vi "Init_For_Programming.vi"(8 "error in (no error)":errorcluster, 10 "board_num":i32, 11 "path in":path) -> (0 "error out":errorcluster, 3 "path out":path)   [LabVIEW 2013, in "SpinAPI-Interface.lvlib"]
uses:
  SpinAPI-Interface.lvlib
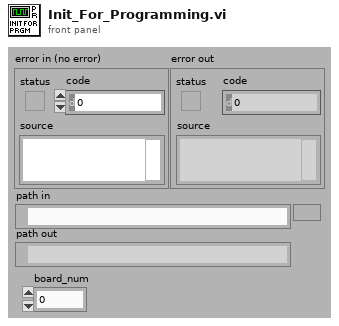
[diagram p1: front panel]
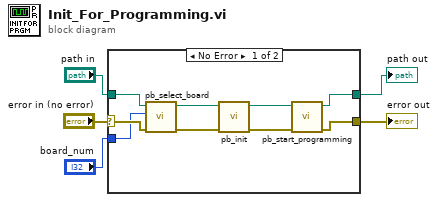
[diagram p0: block diagram]
diagram:
  n1 = case shown="No Error" "error in (no error)" {
    selector: "error in (no error)" -> [w14 w16]
    tunnel: [w11 w16] -> w4
    tunnel: "path in" -> [w7 w15]
    tunnel: [w10 w15] -> w2
    tunnel: "board_num" -> [w6 _]
    frame No Error {
      n2 = call "pb_select_board.vi"("error in (no error)"=w14, "board_num"=w6, "path in"=w7) -> ("error out"=w13:errorcluster, "path out"=w8:path)  [unwired: 7 in]
      n3 = call "pb_init.vi"("error in (no error)"=w13, "path in"=w8) -> ("error out"=w12:errorcluster, "path out"=w9:path)  [unwired: 8 in]
      n4 = call "pb_start_programming.vi"("error in (no error)"=w12, "path in"=w9) -> ("error out"=w11:errorcluster, "path out"=w10:path)  [unwired: 8 in]
    }
    frame Error {
    }
  }
  "error out" <- w4
  "path out" <- w2
